vi "Read Group.vi"(8 "error in (no error)":errorcluster, 10 "Group ID":string, 11 "Configuration Session in":refnum<class "Configuration Session.lvclass">) -> (0 "error out":errorcluster, 1 "value":T1, 3 "Configuration Session out":refnum<class "Configuration Session.lvclass">, 4 "found?":bool)   [LabVIEW 2017, in "DSF Core.lvlib" / "Configuration Session.lvclass"]
doc: "Reads a value associated with a key in a specified section from the configuration data identified by <B>dsf refnum</B>. If the key does not exist, the VI returns the default value. This VI supports multibyte characters in strings. Wire data to the <B>default value</B> input to determine the polymorphic instance to use or manually select the instance."
uses:
  Configuration Session.lvclass
  Typedefs/DSF Timing Info.ctl
  DSF Core.lvlib
  Typedefs/DSF Group Info.ctl
  Typedefs/DSF Direction.ctl
  Typedefs/DSF Timeout Behavior.ctl
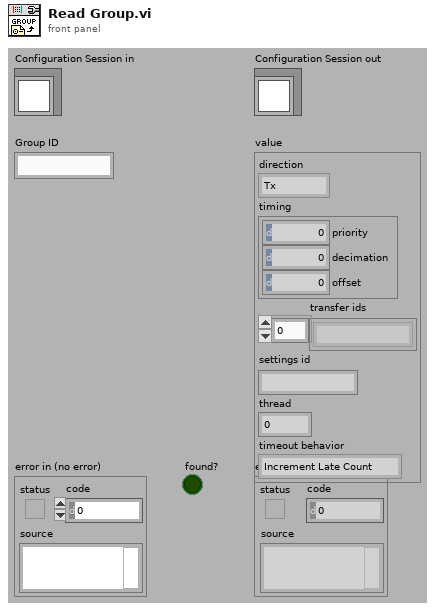
[diagram p1: front panel]
types:
  T1 = typedef "DSF Core.lvlib/DSF Group Info.ctl" = cluster{"direction":T2, "timing":T3, "transfer ids":string[], "settings id":string, "thread":i32, "timeout behavior":T4}
  T2 = typedef "DSF Core.lvlib/DSF Direction.ctl" = enum8{"Tx", "Rx"}
  T3 = typedef "DSF Core.lvlib/DSF Timing Info.ctl" = cluster{"priority":u64, "decimation":u64, "offset":u64}
  T4 = typedef "DSF Core.lvlib/DSF Timeout Behavior.ctl" = enum8{"Increment Late Count", "Throw Error"}
  T5 = typedef "DSF Core.lvlib/Configuration Session.lvclass/DSF Config Data Ref.ctl" = refnum<data-value>
  T6 = typedef "DSF Core.lvlib/Configuration Session.lvclass/DSF Config Data.ctl" = cluster{"path":path, "dirty":bool, "dsf configuration":T7}
  T7 = typedef "DSF Core.lvlib/Configuration Session.lvclass/Internal DSF Configuration.ctl" = cluster{"dsfversion":T8, "version":T8, "framework configuration":T9}
  T8 = typedef "DSF Core.lvlib/DSF Version Info.ctl" = cluster{"major":u32, "minor":u32, "fix":u32, "build":string}
  T9 = typedef "DSF Core.lvlib/Configuration Session.lvclass/DSF Engine Framework JSON Configuration.ctl" = cluster{"Plugins":T10[]}
  T10 = typedef "DSF Core.lvlib/Configuration Session.lvclass/DSF Engine Plugin JSON Configuration.ctl" = cluster{"name":string, "components":string[], "cycle timing":T3, "threads":T11[], "Transfer Groups":T13[], "settings":T12}
  T11 = typedef "DSF Core.lvlib/DSF Engine Plugin Thread Configuration.ctl" = cluster{"buffer converter settings":T12, "transceiver settings":T12, "custom settings":T12, "processor":i32, "priority offset":i16}
  T12 = typedef "DSF Core.lvlib/DSF Settings Info.ctl" = cluster{"key":string, "value":string}[]
  T13 = typedef "DSF Core.lvlib/Configuration Session.lvclass/DSF Engine Transfer Group JSON Configuration.ctl" = cluster{"name":string, "direction":u8, "cycle timing":T3, "thread index":i32, "settings":T12, "Transfers":T14[], "timeout behavior":u8}
  T14 = typedef "DSF Core.lvlib/Configuration Session.lvclass/DSF Engine Transfer JSON Configuration.ctl" = cluster{"name":string, "byte order":u8, "settings":T12, "channels":T15[]}
  T15 = typedef "DSF Core.lvlib/Configuration Session.lvclass/DSF Engine Channel JSON Configuration.ctl" = cluster{"string offset":u64, "string data type":u8, "engine data type":u8, "name":string, "settings":T12, "units":string}
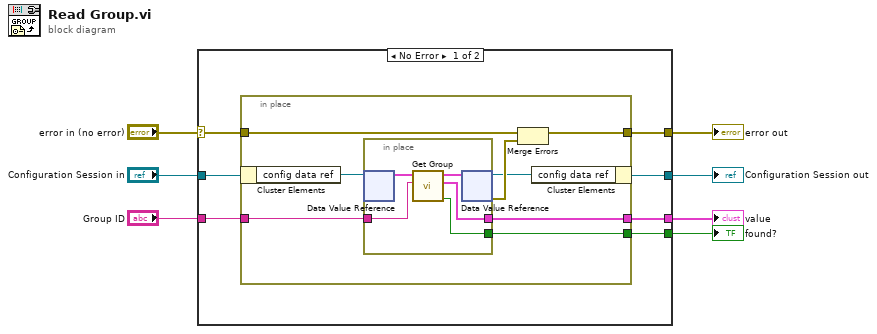
[diagram p0: block diagram]
diagram:
  n1 = case shown="No Error" "error in (no error)" {
    selector: "error in (no error)" -> [w8 w29]
    tunnel: [w14 w29] -> w7
    tunnel: "Group ID" -> [w13 _]
    tunnel: [w12 _] -> w5
    tunnel: [w11 _] -> w4
    tunnel: "Configuration Session in" -> [w10 w28]
    tunnel: [w9 w28] -> w2
    frame No Error {
      n2 = in-place {
        in-place-border: w8 -> [w22]
        in-place-border: [w21] -> w14
        in-place-border: w13 -> [w20]
        in-place-border: [w19] -> w12
        in-place-border: [w18] -> w11
        n3 = in-place-cluster #1(w10) -> ("config data ref"=w16:T5)
        n4 = in-place {
          in-place-border: w20 -> [w27]
          in-place-border: [w26] -> w19
          in-place-border: [w25] -> w18
          n5 = in-place-dvr #2(w16) -> (w24:T6)  [unwired: 1 out]
          n6 = call "Get Group.vi"("id"=w27, "DSF Configuration in"=w24) -> ("exists?"=w25:bool, "info"=w26:T1, "DSF Configuration out"=w23:T6)  [unwired: 6 in, 1 out]
          n7 = in-place-dvr #2(w23) -> (w15:T5, w17:errorcluster)
        }
        n8 = Merge Errors(w22, w17) -> (w21:errorcluster)
        n9 = in-place-cluster #1("config data ref"=w15) -> (w9:refnum<class "Configuration Session.lvclass">)
      }
    }
    frame Error {
    }
  }
  "error out" <- w7
  "found?" <- w4
  "value" <- w5
  "Configuration Session out" <- w2
